vi "Error Query.vi"(8 "error in (no error)":errorcluster, 11 "VISA resource name":refnum<visa-resource-name>) -> (0 "error out":errorcluster, 1 "Error Message":string, 2 "Error Code":i32[](array[numeric]), 3 "VISA resource name out":refnum<visa-resource-name>)   [LabVIEW 2020, in "3458A Basic Driver.lvlib"]
doc: "Queries the instrument for any errors in the instrument's error queue. It will continue to read errors until all errors have been read from the instrument. Any errors will be returned in the Error Out cluster.\n\nNote:\nThis VI is called automatically by most driver VIs so it is not usually necessary to call this in an application."
uses:
  3458A Basic Driver.lvlib
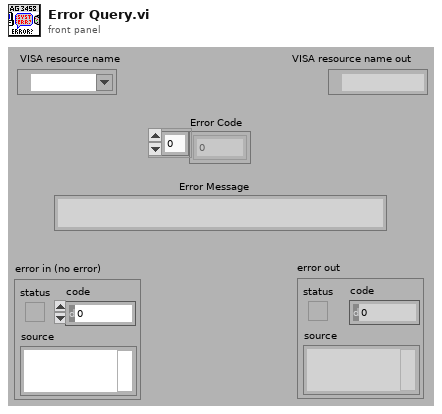
[diagram p1: front panel]
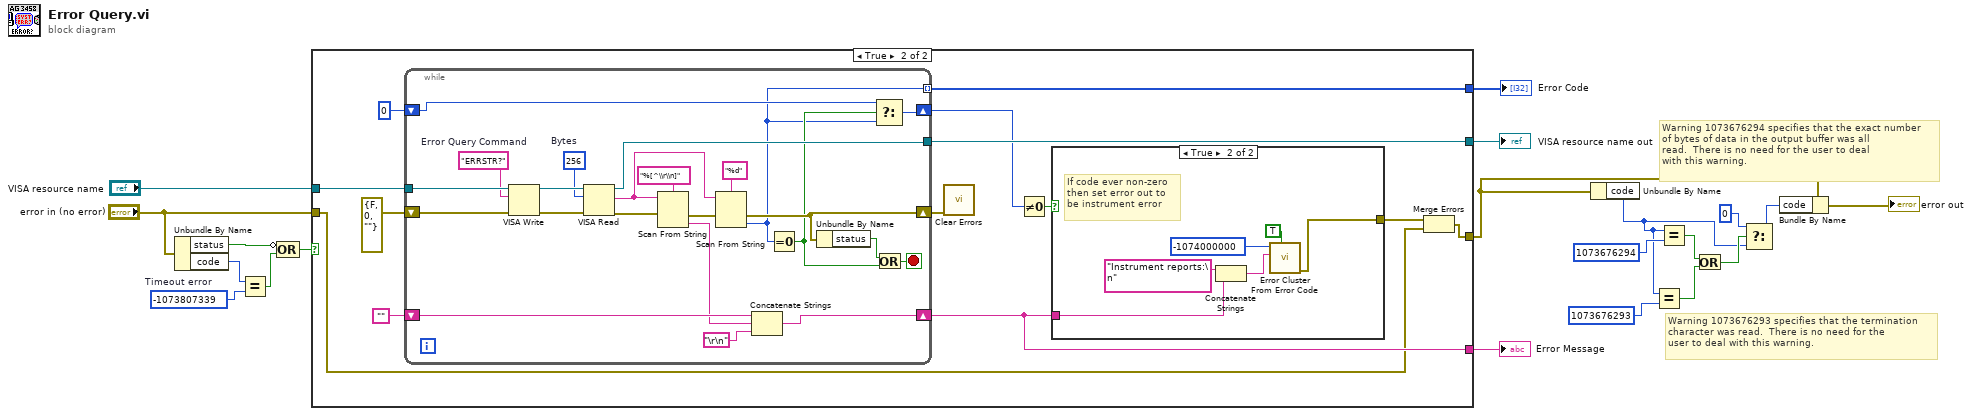
[diagram p0: block diagram]
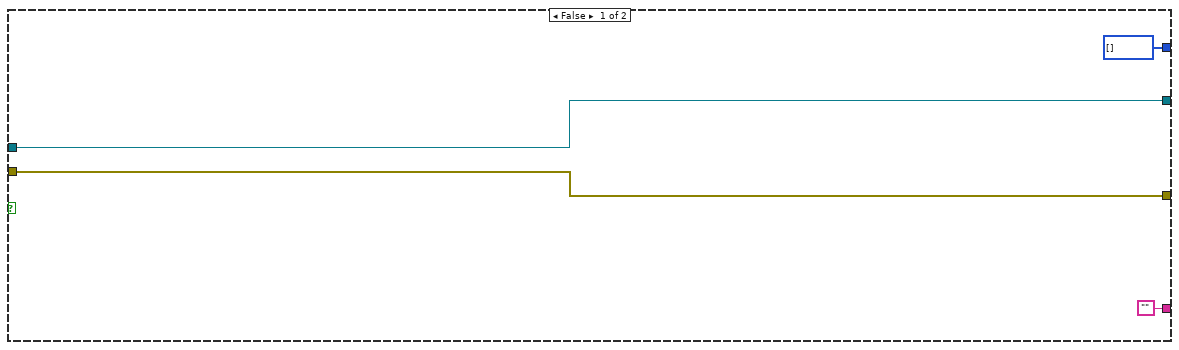
[diagram p2: hidden frame]
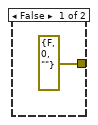
[diagram p3: hidden frame]
diagram:
  w17 = -1073807339  # Timeout error
  # "Warning 1073676293 specifies that the termination \ncharacter was read.  There is no need for the \nuser to deal with this warning."
  # "Warning 1073676294 specifies that the exact number\nof bytes of data in the output buffer was all\nread.  There is no need for the user to deal\nwith this warning."
  n1 = Unbundle By Name("error in (no error)") -> ("status"=w18:bool, "code"=w15:i32)
  n2 = Equal?(x=w15, y=w17) -> (x = y?=w16:bool)
  n3 = Compound Arithmetic op=OR(invert w18, w16) -> (w14:bool)
  n4 = case shown="True" w14 {
    tunnel: [w24 w37] -> w20
    tunnel: "VISA resource name" -> [w24 w36]
    tunnel: "error in (no error)" -> [w23 w26]
    tunnel: [w23 w34] -> w3
    tunnel: ["" w28] -> w13
    tunnel: [i32[] [] w27] -> w12
    frame False {
    }
    frame True {
      n5 = while {
        tunnel: [w67] -> w37
        tunnel: w36 -> [w66]
        shift-right: [w54] -> w28
        shift-left: "" -> [w57]
        shift-right: [w52] -> w29
        shift-left: 0 -> [w53]
        shift-right: [w50] -> w25
        shift-left: errorcluster {"status"=FALSE, "code"=0, "source"=""} ("error in (no error)") -> [w51]
        tunnel: [w45] -> w27 mode=indexing
        stop <- w60 stop-if-true
        w64 = u32 256  # Bytes
        w62 = "ERRSTR?"  # Error Query Command
        n6 = VISA Write(VISA resource name=w66, write buffer=w62, error in (no error)=w51) -> (VISA resource name out=w65:refnum<visa-resource-name>, error out=w63:errorcluster)  [unwired: 1 out]
        n7 = VISA Read(VISA resource name=w65, byte count=w64, error in (no error)=w63) -> (VISA resource name out=w67:refnum<visa-resource-name>, read buffer=w58:string, error out=w49:errorcluster)  [unwired: 1 out]
        n8 = Scan From String(format string="%[^\\r\\n]", input string=w58, error in=w49) -> (error out=w48:errorcluster, output 1=w55:string)  [unwired: 2 in, 2 out]
        n9 = Scan From String(format string="%d", input string=w58, error in=w48) -> (error out=w50:errorcluster, output 1=w45:i32)  [unwired: 2 in, 2 out]
        n10 = Concatenate Strings(w57, w55, "\r\n") -> (w54:string)
        n11 = Equal To 0?(x=w45) -> (x = 0?=w46:bool)
        n12 = Unbundle By Name(w50) -> ("status"=w47:bool)
        n13 = Select(t=w53, s=w46, f=w45) -> (s? t:f=w52:i32)
        n14 = Or(x=w47, y=w46) -> (x .or. y?=w60:bool)
      }
      n15 = call <vilib>:"Clear Errors.vi"("error in (no error)"=w25) -> ()  [unwired: 5 in, 2 out]
      n16 = Not Equal To 0?(x=w29) -> (x != 0?=w32:bool)
      n17 = case shown="True" w32 {
        tunnel: w28 -> [_ w43]
        tunnel: [errorcluster {"status"=FALSE, "code"=0, "source"=""} ("error out") w39] -> w31
        frame False {
        }
        frame True {
          # "If code ever non-zero\nthen set error out to\nbe instrument error"
          n18 = Concatenate Strings("Instrument reports:\n" ("Source"), w43) -> (w40:string)
          n19 = call <vilib>:"Error Cluster From Error Code.vi"("show call chain? (False)"=TRUE, "error message (\"\")"=w40, "error code (0)"=-1074000000 ("Code")) -> ("error out"=w39:errorcluster)  [unwired: 6 in]
        }
      }
      n20 = Merge Errors(w31, w26) -> (w34:errorcluster)
    }
  }
  "VISA resource name out" <- w20
  "Error Message" <- w13
  "Error Code" <- w12
  n21 = Unbundle By Name(w3) -> ("code"=w4:i32)
  n22 = Equal?(x=w4, y=1073676293) -> (x = y?=w7:bool)
  n23 = Equal?(x=w4, y=1073676294) -> (x = y?=w6:bool)
  n24 = Or(x=w6, y=w7) -> (x .or. y?=w5:bool)
  n25 = Select(t=0, s=w5, f=w4) -> (s? t:f=w9:i32)
  n26 = Bundle By Name(cluster=w3, "code"=w9) -> (→"error out":errorcluster)
